vi "BESSY Get Test.vi"() -> ()   [LabVIEW 2011]
uses:
  <userlib>/caLab/sub/caLabGet01.vi
panel:
  in  "PV name (array)":string[](array[string])=["css:sine"]
  out "error out":errorcluster
  out "1st value(number)":dbl[](array[numeric])
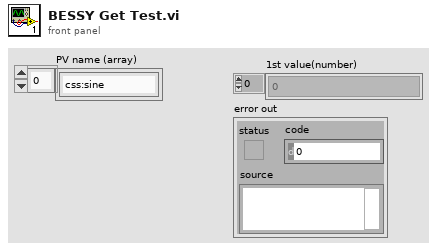
[diagram p1: front panel]
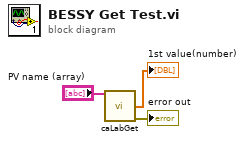
[diagram p0: block diagram]
diagram:
  n1 = call-poly <userlib>:"caLabGet.vi"("PV name (array)"="PV name (array)") -> ("1st value(number)"=→"1st value(number)":dbl[], "error out"=→"error out":errorcluster)  [unwired: 8 in, 5 out]
